vi "Live window-Event handler-linked sliders.vi"(11 "Left/Right":T1) -> ()   [LabVIEW 2013]
uses:
  Typedefs/Left-Right enum.ctl
  Globals/gl_Windows Ctrl refs.vi
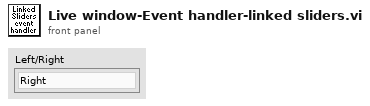
[diagram p1: front panel]
types:
  T1 = typedef "Left-Right enum.ctl" = enum16{"Right", "Left"}
  T2 = typedef "Live window-ctrl refs.ctl" = cluster{"This VI":refnum<vi>, "Pane":refnum<vi>, "Snapshot":refnum<vi>, "Left Image Palette":refnum<vi>, "Right Image Palette":refnum<vi>, "Left Channel":refnum<vi>, "Right Channel":refnum<vi>, "Left image intensity":refnum<vi>, "Right image intensity":refnum<vi>, "Left Image Display":T3, "Right Image Display":T3, "Refresh rate ind (Hz)":refnum<vi>, "Acq rate ind (Hz)":refnum<vi>, "Stop (ind)":refnum<vi>}
  T3 = typedef "Image display ref.ctl" = refnum<vi>
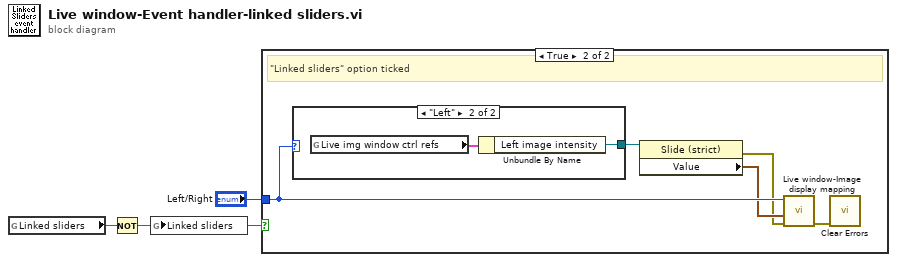
[diagram p0: block diagram]
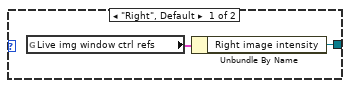
[diagram p3: hidden frame]
diagram:
  n1 = global read "gl_Windows Ctrl refs.vi" "Linked sliders"() -> (w3:bool)
  n2 = Not(x=w3) -> (.not. x?=w2:bool)
  n3 = global write "gl_Windows Ctrl refs.vi" "Linked sliders"(w2) -> ()
  n4 = case shown="True" w2 {
    tunnel: "Left/Right" -> [_ w8]
    frame False {
      # "\"Linked sliders\" option unticked"
    }
    frame True {
      # "\"Linked sliders\" option ticked"
      n5 = case shown="\"Left\"" w8 {
        tunnel: [w9 w11] -> w7
        frame "Right", Default {
          n6 = global read "gl_Windows Ctrl refs.vi" "Live img window ctrl refs"() -> (w10:T2)
          n7 = Unbundle By Name(w10) -> ("Right image intensity"=w9:refnum<vi>)
        }
        frame "Left" {
          n8 = global read "gl_Windows Ctrl refs.vi" "Live img window ctrl refs"() -> (w12:T2)
          n9 = Unbundle By Name(w12) -> ("Left image intensity"=w11:refnum<vi>)
        }
      }
      n10 = property class="Slide (strict)"(reference=w7) -> (error out=w5:errorcluster, "Value"=w6:cluster{i16, i16})  [unwired: 1 in, 1 out]
      n11 = call "Live window-Image display mapping.vi"("error in (no error)"=w5, "Intensity sliders"=w6, "Which image display?"=w8) -> ("error out"=w4:errorcluster)  [unwired: 8 in]
      n12 = call <vilib>:"Clear Errors.vi"("error in (no error)"=w4) -> ()  [unwired: 6 in, 1 out]
    }
  }
